vi "write_mat_file_2020.vi"   [LabVIEW 2020]
uses:
  <vilib>/Platform/storage/Storage.llb/usiSequenceRepresentation.ctl
  <vilib>/Platform/storage/lvStorage.llb/_defaultFilePath.vi
  <vilib>/Platform/storage/lvStorage.llb/_openStorageWithRootAutoDetect.vi
  <vilib>/Platform/storage/lvStorage.llb/xStorage/xStorageSupp/ErrorOut.vi
  <vilib>/Platform/storage/lvStorage.llb/_createOrGetExplicitChildObject.vi
  <vilib>/Platform/storage/lvStorage.llb/_createOrGetByNameExplicitChildObject.vi
  <vilib>/Platform/storage/lvStorage.llb/_saveFloat64Channel.vi
  <vilib>/Platform/storage/Storage.llb/Get Object Info.vi
  <vilib>/Platform/storage/Storage.llb/__closeStorageFromObject.vi
  <vilib>/Platform/storage/lvStorage.llb/xStorage/Open Data Storage/Open Data Storage.xnode
  <vilib>/Platform/storage/lvStorage.llb/xStorage/Write Data/Write Data.xnode
  <vilib>/Platform/storage/lvStorage.llb/xStorage/Close Data Storage/Close Data Storage.xnode
types:
  T1 = enum16{"Append values", "Replace values at index", "Replace all values"}
  T2 = enum16{"open", "open or create", "create or replace", "create", "open (read only)"}
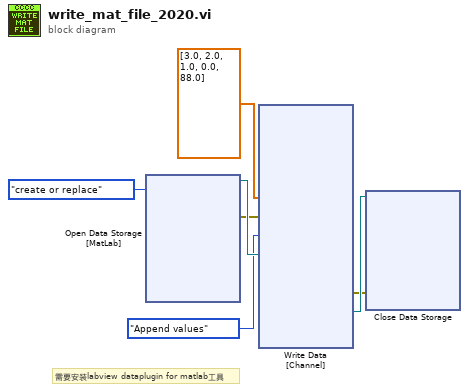
[diagram p0: block diagram]
diagram:
  # "需要安装labview dataplugin for matlab工具"
  n1 = xnode "Open Data Storage\n[MatLab]"("function (open:0)"=T2."create or replace") -> ("storage refnum (file)"=w7:refnum<k20>, "error out"=w4:errorcluster)  [unwired: 4 in, 1 out]
  n2 = xnode "Write Data\n[Channel]"("Signal"=dbl[] [3.0, 2.0, 1.0, 0.0, 88.0], "error in"=w4, "append / replace (append data values)"=T1."Append values", "storage refnum (file)"=w7) -> ("error out"=w5:errorcluster, "storage refnum (file) out"=w6:refnum<k20>)  [unwired: 1 in, 1 out]
  n3 = xnode "Close Data Storage\n"("error in (no error)"=w5, "storage refnum (file)"=w6) -> ()  [unwired: 2 out]
